vi "log analysis_gps.vi"() -> ()   [LabVIEW 2019] (continued)
0.3968,0.2930,0.5072,0.1078,0.0917,0.0751,0.1476,0.1496,5.0204,0f000001,0*5136ca20\n\t", "INSPVAXA,USB3,0,44.0,FINESTEERING,2107,282107.450,02000000,471d,15824;INS_ALIGNMENT_COMPLETE,INS_RTKFIXED,37.37095551506,126.72370946213,8.7227,22.3000,-0.1464,0.2502,0.0156,-0.936172746,1.990543984,117.627917664,0.3961,0.2929,0.5071,0.1075,0.0916,0.0751,0.1476,0.1496,5.0204,0f000001,0*d8872792\n\t", "INSPVAXA,USB3,0,44.0,FINESTEERING,2107,282107.950,02000000,471d,15824;INS_ALIGNMENT_COMPLETE,INS_RTKFIXED,37.37095481415,126.72371079890,8.7282,22.3000,-0.1478,0.2544,0.0132,-0.866251632,1.815335912,117.612256060,0.3961,0.2929,0.5071,0.1075,0.0916,0.0751,0.1476,0.1496,5.0204,0f000001,0*57d0bda5\n\t", "INSPVAXA,USB3,0,47.5,FINESTEERING,2107,282108.450,02000000,471d,15824;INS_ALIGNMENT_COMPLETE,INS_RTKFIXED,37.37095411436,126.72371215377,8.7320,22.3000,-0.1500,0.2481,0.0140,-1.024789721,1.612981826,117.661458987,0.3956,0.2928,0.5070,0.1077,0.0917,0.0751,0.1475,0.1496,5.0202,0f000001,0*a0675bbc\n\t", "INSPVAXA,USB3,0,47.5,FINESTEERING,2107,282108.950,02000000,471d,15824;INS_ALIGNMENT_COMPLETE,INS_RTKFIXED,37.37095342524,126.72371347450,8.7365,22.3000,-0.1464,0.2522,0.0087,-1.211194385,1.652387786,117.710321786,0.3956,0.2928,0.5070,0.1077,0.0917,0.0751,0.1475,0.1496,5.0202,0f000001,0*fbbb71e9\n\t", "INSPVAXA,USB3,0,48.0,FINESTEERING,2107,282109.450,02000000,471d,15824;INS_ALIGNMENT_COMPLETE,INS_RTKFIXED,37.37095274133,126.72371479106,8.7424,22.3000,-0.1538,0.2512,0.0057,-1.183703798,1.673883858,117.732528128,0.3953,0.2928,0.5071,0.1077,0.0917,0.0751,0.1475,0.1496,5.0195,0f000001,0*a98a5245\n\t", "INSPVAXA,USB3,0,48.0,FINESTEERING,2107,282109.950,02000000,471d,15824;INS_ALIGNMENT_COMPLETE,INS_RTKFIXED,37.37095203304,126.72371616104,8.7487,22.3000,-0.1514,0.2528,0.0147,-1.036882261,1.559922655,117.777953155,0.3953,0.2928,0.5071,0.1077,0.0917,0.0751,0.1475,0.1496,5.0195,0f000001,0*d50cd7f7\n\t", "INSPVAXA,USB3,0,48.5,FINESTEERING,2107,282110.450,02000000,471d,15824;INS_ALIGNMENT_COMPLETE,INS_RTKFIXED,37.37095133527,126.72371748883,8.7530,22.3000,-0.1494,0.2469,0.0119,-1.026348823,1.537323059,117.877652049,0.3951,0.2928,0.5070,0.1077,0.0917,0.0751,0.1475,0.1496,5.0182,0f000001,0*ecbd9d89\n\t", "INSPVAXA,USB3,0,48.5,FINESTEERING,2107,282110.950,02000000,471d,15824;INS_ALIGNMENT_COMPLETE,INS_RTKFIXED,37.37095063141,126.72371883736,8.7567,22.3000,-0.1443,0.2312,0.0129,-1.128303497,1.542678809,118.026662583,0.3951,0.2928,0.5070,0.1077,0.0917,0.0751,0.1475,0.1496,5.0182,0f000001,0*daaca067\n\t", "INSPVAXA,USB3,0,46.0,FINESTEERING,2107,282111.450,02000000,471d,15824;INS_ALIGNMENT_COMPLETE,INS_RTKFIXED,37.37094994978,126.72372015306,8.7620,22.3000,-0.1561,0.2454,0.0089,-1.155550094,1.466986679,118.115120191,0.3996,0.2955,0.5135,0.1085,0.0924,0.0757,0.1476,0.1497,5.0168,0f000001,0*9d755c1d\n\t", "INSPVAXA,USB3,0,46.0,FINESTEERING,2107,282111.950,02000000,471d,15824;INS_ALIGNMENT_COMPLETE,INS_RTKFIXED,37.37094924686,126.72372148621,8.7667,22.3000,-0.1592,0.2411,0.0080,-1.003376747,1.533507787,118.272208873,0.3996,0.2955,0.5135,0.1085,0.0924,0.0757,0.1476,0.1497,5.0168,0f000001,0*68376ab3\n\t", "INSPVAXA,USB3,0,47.5,FINESTEERING,2107,282113.450,02000000,471d,15824;INS_ALIGNMENT_COMPLETE,INS_RTKFIXED,37.37094709383,126.72372548494,8.7822,22.3000,-0.1691,0.2475,0.0112,-0.824972405,1.586356961,118.983770593,0.4030,0.2950,0.5178,0.1084,0.0922,0.0757,0.1475,0.1497,5.0138,0f000001,0*59439988\n\t", "INSPVAXA,USB3,0,51.5,FINESTEERING,2107,282114.950,02000000,471d,15824;INS_ALIGNMENT_COMPLETE,INS_RTKFIXED,37.37094483188,126.72372951627,8.7947,22.3000,-0.1730,0.2314,0.0140,-0.653922567,1.323648308,119.738020967,0.4016,0.2936,0.5159,0.1080,0.0922,0.0755,0.1474,0.1496,5.0125,0f000001,0*093f9180\n\t", "INSPVAXA,USB3,0,50.5,FINESTEERING,2107,282115.450,02000000,471d,15824;INS_ALIGNMENT_COMPLETE,INS_RTKFIXED,37.37094409692,126.72373081199,8.8000,22.3000,-0.1872,0.2511,0.0165,-0.607846314,1.413014132,119.977031024,0.3998,0.2929,0.5140,0.1075,0.0920,0.0753,0.1474,0.1495,5.0103,0f000001,0*d87b3f60\n\t", "INSPVAXA,USB3,0,50.5,FINESTEERING,2107,282115.950,02000000,471d,15824;INS_ALIGNMENT_COMPLETE,INS_RTKFIXED,37.37094333872,126.72373213439,8.8049,22.3000,-0.1750,0.2376,0.0100,-0.458555016,1.505006128,120.195242243,0.3998,0.2929,0.5140,0.1075,0.0920,0.0753,0.1474,0.1495,5.0103,0f000001,0*9085454d\n\t", "INSPVAXA,USB3,0,47.5,FINESTEERING,2107,282116.450,02000000,471d,15824;INS_ALIGNMENT_COMPLETE,INS_RTKFIXED,37.37094260633,126.72373343529,8.8096,22.3000,-0.1820,0.2326,0.0074,-0.394320906,1.730091512,120.395772522,0.3983,0.2926,0.5122,0.1073,0.0921,0.0752,0.1473,0.1495,5.0085,0f000001,0*0af836cc\n\t", "INSPVAXA,USB3,0,47.5,FINESTEERING,2107,282116.950,02000000,471d,15824;INS_ALIGNMENT_COMPLETE,INS_RTKFIXED,37.37094186601,126.72373474956,8.8141,22.3000,-0.1805,0.2419,0.0176,-0.396545512,1.701319201,120.653391507,0.3983,0.2926,0.5122,0.1073,0.0921,0.0752,0.1473,0.1495,5.0085,0f000001,0*1c5a80aa\n\t", "INSPVAXA,USB3,0,50.0,FINESTEERING,2107,282117.450,02000000,471d,15824;INS_ALIGNMENT_COMPLETE,INS_RTKFIXED,37.37094111146,126.72373605556,8.8178,22.3000,-0.1868,0.2460,0.0165,-0.381592646,1.647549493,120.846709462,0.3974,0.2926,0.5106,0.1073,0.0921,0.0751,0.1472,0.1494,5.0066,0f000001,0*ba01e3a8\n\t", "INSPVAXA,USB3,0,50.0,FINESTEERING,2107,282117.950,02000000,471d,15824;INS_ALIGNMENT_COMPLETE,INS_RTKFIXED,37.37094033819,126.72373738098,8.8215,22.3000,-0.1807,0.2431,0.0157,-0.357927005,1.593594515,120.982465037,0.3974,0.2926,0.5106,0.1073,0.0921,0.0751,0.1472,0.1494,5.0066,0f000001,0*473a97aa\n\t", "INSPVAXA,USB3,0,47.0,FINESTEERING,2107,282118.450,02000000,471d,15824;INS_ALIGNMENT_COMPLETE,INS_RTKFIXED,37.37093956964,126.72373870165,8.8242,22.3000,-0.1812,0.2503,0.0145,-0.278070640,1.434405224,121.098239314,0.3976,0.2926,0.5095,0.1073,0.0920,0.0750,0.1472,0.1494,5.0051,0f000001,0*4b2331c4\n\t", "INSPVAXA,USB3,0,47.0,FINESTEERING,2107,282118.950,02000000,471d,15824;INS_ALIGNMENT_COMPLETE,INS_RTKFIXED,37.37093879764,126.72374003076,8.8271,22.3000,-0.1824,0.2531,0.0181,-0.239679007,1.415709773,121.121487507,0.3976,0.2926,0.5095,0.1073,0.0920,0.0750,0.1472,0.1494,5.0051,0f000001,0*31152a6b\n\t", "INSPVAXA,USB3,0,51.0,FINESTEERING,2107,282119.950,02000000,471d,15824;INS_ALIGNMENT_COMPLETE,INS_RTKFIXED,37.37093727154,126.72374264951,8.8356,22.3000,-0.1820,0.2425,0.0126,-0.263751885,1.526286422,121.184806545,0.3974,0.2926,0.5086,0.1074,0.0920,0.0750,0.1471,0.1494,5.0040,0f000001,0*c7b594c4\n\t", "INSPVAXA,USB3,0,49.5,FINESTEERING,2107,282121.950,02000000,471d,15824;INS_ALIGNMENT_COMPLETE,INS_RTKFIXED,37.37093422508,126.72374790381,8.8513,22.3000,-0.1769,0.2415,0.0095,-0.361327537,1.582717888,121.199299020,0.3976,0.2927,0.5074,0.1074,0.0918,0.0750,0.1470,0.1494,5.0032,0f000001,0*bd59e65f\n\t", "INSPVAXA,USB3,0,51.5,FINESTEERING,2107,282122.950,02000000,471d,15824;INS_ALIGNMENT_COMPLETE,INS_RTKFIXED,37.37093271089,126.72375052599,8.8596,22.3000,-0.1652,0.2321,0.0060,-0.281890113,1.847721307,121.184840630,0.3974,0.2927,0.5070,0.1074,0.0918,0.0750,0.1469,0.1494,5.0040,0f000001,0*3de7c804\n\t", "INSPVAXA,USB3,0,51.0,FINESTEERING,2107,282151.500,02000000,471d,15824;INS_ALIGNMENT_COMPLETE,INS_RTKFIXED,37.37088960505,126.72382499990,9.1778,22.3000,-0.1858,0.2425,0.0007,-0.584217482,1.708777597,119.499420224,0.4348,0.2933,0.5266,0.1137,0.0921,0.0762,0.1458,0.1498,5.0245,0f000001,0*a137cdab\n\t", "INSPVAXA,USB3,0,46.5,FINESTEERING,2107,282153.500,02000000,471d,15824;INS_ALIGNMENT_COMPLETE,INS_RTKFIXED,37.37088668027,126.72383030308,9.1844,22.3000,-0.1846,0.2433,-0.0063,-0.490970731,1.271254139,120.414068071,0.4478,0.2935,0.5351,0.1145,0.0921,0.0767,0.1457,0.1497,5.0277,0f000001,0*2a0513c3\n\t", "INSPVAXA,USB3,0,47.0,FINESTEERING,2107,282154.500,02000000,471d,15824;INS_ALIGNMENT_COMPLETE,INS_RTKFIXED,37.37088518540,126.72383296501,9.1848,22.3000,-0.1849,0.2389,0.0033,-0.578089293,1.343840193,120.921980586,0.4509,0.2935,0.5383,0.1145,0.0921,0.0767,0.1457,0.1497,5.0293,0f000001,0*6c2251c0\n\t", "INSPVAXA,USB3,0,49.5,FINESTEERING,2107,282156.000,02000000,471d,15824;INS_ALIGNMENT_COMPLETE,INS_RTKFIXED,37.37088292743,126.72383688922,9.1933,22.3000,-0.1804,0.2249,-0.0069,-0.526000833,1.617795510,121.650926042,0.4526,0.2935,0.5409,0.1144,0.0920,0.0768,0.1457,0.1496,5.0309,0f000001,0*7b06a300\n\t", "INSPVAXA,USB3,0,48.5,FINESTEERING,2107,282156.500,02000000,471d,15824;INS_ALIGNMENT_COMPLETE,INS_RTKFIXED,37.37088217363,126.72383817131,9.1964,22.3000,-0.1807,0.2394,-0.0085,-0.574321613,1.643212102,121.914347439,0.4534,0.2936,0.5427,0.1143,0.0921,0.0768,0.1456,0.1496,5.0325,0f000001,0*15ca3725\n\t", "INSPVAXA,USB3,0,48.5,FINESTEERING,2107,282157.000,02000000,471d,15824;INS_ALIGNMENT_COMPLETE,INS_RTKFIXED,37.37088140399,126.72383945930,9.1993,22.3000,-0.1862,0.2446,-0.0064,-0.600405217,1.496036608,122.180467270,0.4534,0.2936,0.5427,0.1143,0.0921,0.0768,0.1456,0.1496,5.0325,0f000001,0*c5e5c6e3\n\t", "INSPVAXA,USB3,0,45.5,FINESTEERING,2107,282158.500,02000000,471d,15824;INS_ALIGNMENT_COMPLETE,INS_RTKFIXED,37.37087907876,126.72384326761,9.2104,22.3000,-0.1767,0.2291,0.0108,-0.395230088,1.351210238,122.917750135,0.4537,0.2937,0.5451,0.1144,0.0921,0.0768,0.1456,0.1495,5.0357,0f000001,0*07daf6c2\n\t", "INSPVAXA,USB3,0,45.5,FINESTEERING,2107,282159.000,02000000,471d,15824;INS_ALIGNMENT_COMPLETE,INS_RTKFIXED,37.37087827658,126.72384453527,9.2150,22.3000,-0.1825,0.2336,0.0127,-0.281125763,1.400376320,123.162742277,0.4537,0.2937,0.5451,0.1144,0.0921,0.0768,0.1456,0.1495,5.0357,0f000001,0*5700aa0a\n\t", "INSPVAXA,USB3,0,48.5,FINESTEERING,2107,282161.000,02000000,471d,15824;INS_ALIGNMENT_COMPLETE,INS_RTKFIXED,37.37087514986,126.72384964420,9.2386,22.3000,-0.1845,0.2318,0.0206,-0.134311793,1.526790970,123.449672080,0.4533,0.2938,0.5460,0.1147,0.0921,0.0768,0.1455,0.1496,5.0387,0f000001,0*1e397fdc\n\t", "INSPVAXA,USB3,0,49.0,FINESTEERING,2107,282162.000,02000000,471d,15824;INS_ALIGNMENT_COMPLETE,INS_RTKFIXED,37.37087356615,126.72385221886,9.2529,22.3000,-0.1851,0.2394,-0.0036,-0.080021339,1.630723538,123.455447603,0.4532,0.2939,0.5462,0.1148,0.0921,0.0768,0.1454,0.1496,5.0402,0f000001,0*5854c212\n\t", "INSPVAXA,USB3,0,51.0,FINESTEERING,2107,282162.500,02000000,471d,15824;INS_ALIGNMENT_COMPLETE,INS_RTKFIXED,37.37087276598,126.72385350535,9.2616,22.3000,-0.1911,0.2293,0.0115,-0.073182754,1.698964868,123.450820933,0.4532,0.2939,0.5462,0.1150,0.0921,0.0768,0.1454,0.1496,5.0417,0f000001,0*35a5fbef\n\t", "INSPVAXA,USB3,0,51.0,FINESTEERING,2107,282163.000,02000000,471d,15824;INS_ALIGNMENT_COMPLETE,INS_RTKFIXED,37.37087198418,126.72385476769,9.2713,22.3000,-0.1886,0.2265,0.0207,-0.163897307,1.756288597,123.387194402,0.4532,0.2939,0.5462,0.1150,0.0921,0.0768,0.1454,0.1496,5.0417,0f000001,0*f7296fb4\n\t", "INSPVAXA,USB3,0,50.0,FINESTEERING,2107,282163.500,02000000,471d,15824;INS_ALIGNMENT_COMPLETE,INS_RTKFIXED,37.37087116734,126.72385603736,9.2795,22.3000,-0.1822,0.2264,0.0180,-0.228587283,1.950230328,123.198406451,0.4532,0.2939,0.5462,0.1150,0.0921,0.0768,0.1454,0.1496,5.0417,0f000001,0*1ae1e07b\n\t", "INSPVAXA,USB3,0,50.0,FINESTEERING,2107,282164.000,02000000,471d,15824;INS_ALIGNMENT_COMPLETE,INS_RTKFIXED,37.37087034978,126.72385731621,9.2879,22.3000,-0.1896,0.2295,0.0123,-0.289631727,1.840561194,122.888440752,0.4532,0.2939,0.5462,0.1150,0.0921,0.0768,0.1454,0.1496,5.0417,0f000001,0*056b33eb\n\t", "INSPVAXA,USB3,0,49.5,FINESTEERING,2107,282164.500,02008000,471d,15824;INS_ALIGNMENT_COMPLETE,INS_RTKFIXED,37.37086961397,126.72385855899,9.2957,22.3000,-0.1725,0.2178,0.0037,-0.245083318,1.835832496,122.519490120,0.5068,0.3317,0.5928,0.1224,0.0977,0.0793,0.1462,0.1507,5.0448,0f000001,0*242e4928\n\t", "INSPVAXA,USB3,0,49.5,FINESTEERING,2107,282165.000,02008000,471d,15824;INS_ALIGNMENT_COMPLETE,INS_RTKFIXED,37.37086887660,126.72385979146,9.3053,22.3000,-0.1797,0.2392,0.0086,-0.083873160,1.728047221,122.128251979,0.5068,0.3317,0.5928,0.1224,0.0977,0.0793,0.1462,0.1507,5.0448,0f000001,0*7f8693c0\n\t", "INSPVAXA,USB3,0,50.0,FINESTEERING,2107,282165.500,02008000,471d,15824;INS_ALIGNMENT_COMPLETE,INS_RTKFIXED,37.37086811316,126.72386104230,9.3143,22.3000,-0.1621,0.2209,0.0106,0.024861587,1.649578148,121.656445407,0.4863,0.3145,0.5830,0.1190,0.0946,0.0782,0.1458,0.1502,5.0461,0f000001,0*34f23d42\n\t", "INSPVAXA,USB3,0,50.0,FINESTEERING,2107,282166.000,02008000,471d,15824;INS_ALIGNMENT_COMPLETE,INS_RTKFIXED,37.37086751829,126.72386195729,9.3219,22.3000,-0.0093,-0.0451,0.0007,-0.021903893,1.492441336,121.617580212,0.4863,0.3145,0.5830,0.1190,0.0946,0.0782,0.1458,0.1502,5.0461,0f000001,0*e5b24ae3\n\t", "INSPVAXA,USB3,0,48.5,FINESTEERING,2107,282166.500,02008000,471d,15824;INS_ALIGNMENT_COMPLETE,INS_RTKFIXED,37.37086745954,126.72386181526,9.3232,22.3000,-0.0268,-0.0236,0.0089,-0.043372783,1.566427448,121.563343894,0.4732,0.3047,0.5748,0.1189,0.0947,0.0774,0.1456,0.1500,5.0475,0f000001,0*3570ed60\n\t", "INSPVAXA,USB3,0,48.5,FINESTEERING,2107,282167.000,02008000,471d,15824;INS_ALIGNMENT_COMPLETE,INS_RTKFIXED,37.37086722262,126.72386202898,9.3264,22.3000,-0.1700,0.2085,0.0159,-0.059764704,1.681922525,121.297414016,0.4732,0.3047,0.5748,0.1189,0.0947,0.0774,0.1456,0.1500,5.0475,0f000001,0*686f29fa\n\t", "INSPVAXA,USB3,0,51.0,FINESTEERING,2107,282167.500,02008000,471d,15824;INS_ALIGNMENT_COMPLETE,INS_RTKFIXED,37.37086635075,126.72386343693,9.3355,22.3000,-0.1343,0.1551,0.0138,-0.191041256,1.725233794,121.448181107,0.4732,0.3047,0.5748,0.1189,0.0947,0.0774,0.1456,0.1500,5.0475,0f000001,0*c09661b1\n\t", "INSPVAXA,USB3,0,51.0,FINESTEERING,2107,282168.000,02008000,471d,15824;INS_ALIGNMENT_COMPLETE,INS_RTKFIXED,37.37086554629,126.72386469627,9.3449,22.3000,-0.1443,0.1947,0.0175,-0.193885511,1.717406727,121.172307594,0.4732,0.3047,0.5748,0.1189,0.0947,0.0774,0.1456,0.1500,5.0475,0f000001,0*05ac97bf\n\t", "INSPVAXA,USB3,0,51.0,FINESTEERING,2107,282168.500,02000000,471d,15824;INS_ALIGNMENT_COMPLETE,INS_RTKFIXED,37.37086484906,126.72386602613,9.3508,22.3000,-0.1684,0.2118,0.0292,-0.052015142,1.767687292,120.756942814,0.5200,0.3367,0.6136,0.1257,0.1009,0.0794,0.1465,0.1509,5.0427,0f000001,0*74b10fb1\n\t", "INSPVAXA,USB3,0,51.0,FINESTEERING,2107,282169.000,02000000,471d,15824;INS_ALIGNMENT_COMPLETE,INS_RTKFIXED,37.37086415822,126.72386736868,9.3575,22.3000,-0.1707,0.2211,0.0151,0.018670150,1.718273405,120.397652354,0.5200,0.3367,0.6136,0.1257,0.1009,0.0794,0.1465,0.1509,5.0427,0f000001,0*7f0a75ca\n\t", "INSPVAXA,USB3,0,46.0,FINESTEERING,2107,282169.500,02000000,471d,15824;INS_ALIGNMENT_COMPLETE,INS_RTKFIXED,37.37086344397,126.72386871844,9.3630,22.3000,-0.1742,0.2275,0.0011,-0.016191041,1.633927809,119.983496476,0.4955,0.3175,0.5974,0.1215,0.0969,0.0780,0.1460,0.1504,5.0326,0f000001,0*70440743\n\t", "DUALANTENNAHEADINGA,USB3,0,46.0,FINESTEERING,2107,282170.000,02000000,d426,15824;INSUFFICIENT_OBS,NONE,0.000000000,0.000000000,0.000000000,0.0,0.000000000,0.000000000,\"\",0,0,0,0,00,00,00,00*d9bd9ff7\n\t", "INSPVAXA,USB3,0,49.5,FINESTEERING,2107,282170.500,02000000,471d,15824;INS_ALIGNMENT_COMPLETE,INS_RTKFIXED,37.37086196149,126.72387133593,9.3775,22.3000,-0.1638,0.2319,0.0101,-0.134678922,1.597363801,119.344832889,0.4955,0.3175,0.5974,0.1215,0.0969,0.0780,0.1460,0.1504,5.0326,0f000001,0*0ad13adf\n\t", "INSPVAXA,USB3,0,49.5,FINESTEERING,2107,282171.000,02000000,471d,15824;INS_ALIGNMENT_COMPLETE,INS_RTKFIXED,37.37086118756,126.72387260380,9.3866,22.3000,-0.1780,0.2223,0.0226,-0.237576400,1.617402983,119.136823599,0.4955,0.3175,0.5974,0.1215,0.0969,0.0780,0.1460,0.1504,5.0326,0f000001,0*d3c2583e\n\t", "DUALANTENNAHEADINGA,USB3,0,52.5,FINESTEERING,2107,282171.500,02000000,d426,15824;SOL_COMPUTED,L1_FLOAT,-1.000000000,212.575851440,56.383117676,0.0,44.713680267,134.992919922,\"631T\",11,5,5,5,04,00,20,02*bb8370c9\n\t", "INSPVAXA,USB3,0,52.5,FINESTEERING,2107,282172.000,02000000,471d,15824;INS_ALIGNMENT_COMPLETE,INS_RTKFIXED,37.37085961658,126.72387509904,9.4055,22.3000,-0.1866,0.2197,0.0120,-0.164173617,1.908755927,118.881251858,0.4955,0.3175,0.5974,0.1215,0.0969,0.0780,0.1460,0.1504,5.0326,0f000001,0*7b1cb490\n\t", "DUALANTENNAHEADINGA,USB3,0,51.0,FINESTEERING,2107,282172.500,02008000,d426,15824;SOL_COMPUTED,NARROW_FLOAT,-1.000000000,128.001327515,-71.010498047,0.0,360.000000000,151.438781738,\"631T\",13,7,7,5,04,00,20,03*76c36059\n\t", "INSPVAXA,USB3,0,51.0,FINESTEERING,2107,282173.000,02008000,471d,15824;INS_ALIGNMENT_COMPLETE,INS_RTKFIXED,37.37085833527,126.72387797741,9.4066,22.3000,-0.1810,0.2279,0.0198,-0.406869052,2.030704243,118.923772886,0.5770,0.3723,0.6754,0.1336,0.1058,0.0814,0.1476,0.1521,5.0145,0f000001,0*4f67786d\n\t", "INSPVAXA,USB3,0,51.0,FINESTEERING,2107,282173.500,02008000,471d,15824;INS_ALIGNMENT_COMPLETE,INS_RTKFIXED,37.37085763620,126.72387935658,9.4103,22.3000,-0.1736,0.2330,0.0207,-0.517446305,1.873578132,118.931812586,0.5249,0.3329,0.6407,0.1266,0.1009,0.0786,0.1470,0.1512,5.0071,0f000001,0*4ebf01a6\n\t", "DUALANTENNAHEADINGA,USB3,0,51.0,FINESTEERING,2107,282174.000,02008000,d426,15824;SOL_COMPUTED,NARROW_FLOAT,-1.000000000,123.069808960,-65.629364014,0.0,360.000000000,180.000000000,\"631T\",16,6,6,5,04,00,20,03*92b169c2\n\t", "DUALANTENNAHEADINGA,USB3,0,49.0,FINESTEERING,2107,282174.500,02008000,d426,15824;SOL_COMPUTED,NARROW_FLOAT,-1.000000000,124.551315308,-68.632659912,0.0,360.000000000,180.000000000,\"631T\",16,7,7,5,04,00,20,03*6a9e420e\n\t", "INSPVAXA,USB3,0,49.0,FINESTEERING,2107,282175.000,02008000,471d,15824;INS_ALIGNMENT_COMPLETE,INS_RTKFIXED,37.37085549477,126.72388337891,9.4209,22.3000,-0.1860,0.2237,0.0201,-0.564638995,1.417085276,119.025707092,0.4961,0.3139,0.6151,0.1240,0.1000,0.0771,0.1467,0.1509,5.0036,0f000001,0*2746038f\n\t", "INSPVAXA,USB3,0,50.0,FINESTEERING,2107,282175.500,02008000,471d,15824;INS_ALIGNMENT_COMPLETE,INS_RTKFIXED,37.37085479315,126.72388469742,9.4248,22.3000,-0.1822,0.2271,0.0141,-0.513806522,1.414717204,119.104354508,0.4791,0.3046,0.5957,0.1234,0.0999,0.0764,0.1464,0.1507,5.0029,0f000001,0*e3204e40\n\t", "INSPVAXA,USB3,0,50.0,FINESTEERING,2107,282176.000,02008000,471d,15824;INS_ALIGNMENT_COMPLETE,INS_RTKFIXED,37.37085410326,126.72388599341,9.4283,22.3000,-0.1760,0.2106,0.0151,-0.605541417,1.454743259,119.281713752,0.4791,0.3046,0.5957,0.1234,0.0999,0.0764,0.1464,0.1507,5.0029,0f000001,0*bcb93fc8\n\t", "DUALANTENNAHEADINGA,USB3,0,48.5,FINESTEERING,2107,282176.500,02000000,d426,15824;SOL_COMPUTED,NARROW_FLOAT,-1.000000000,134.305130005,-57.419616699,0.0,360.000000000,180.000000000,\"631T\",18,6,6,5,04,00,20,03*ffb18b5f\n\t", "DUALANTENNAHEADINGA,USB3,0,48.5,FINESTEERING,2107,282177.000,02000000,d426,15824;SOL_COMPUTED,NARROW_FLOAT,-1.000000000,135.311111450,-57.297637939,0.0,360.000000000,180.000000000,\"631T\",18,6,6,5,04,00,20,03*ffb49dec\n\t", "INSPVAXA,USB3,0,48.0,FINESTEERING,2107,282177.500,02000000,471d,15824;INS_ALIGNMENT_COMPLETE,INS_RTKFIXED,37.37085188860,126.72389002075,9.4437,22.3000,-0.1883,0.2420,0.0164,-0.505003517,1.427423679,120.083460934,0.4645,0.2990,0.5702,0.1231,0.0988,0.0761,0.1455,0.1502,5.0044,0f000001,0*390fa34e\n\t", "INSPVAXA,USB3,0,48.0,FINESTEERING,2107,282178.000,02000000,471d,15824;INS_ALIGNMENT_COMPLETE,INS_RTKFIXED,37.37085112539,126.72389137243,9.4485,22.3000,-0.1737,0.2237,0.0239,-0.447467240,1.418285202,120.360306359,0.4645,0.2990,0.5702,0.1231,0.0988,0.0761,0.1455,0.1502,5.0044,0f000001,0*ee66b8d3\n\t", "DUALANTENNAHEADINGA,USB3,0,48.5,FINESTEERING,2107,282178.500,02000000,d426,15824;SOL_COMPUTED,L1_FLOAT,-1.000000000,214.039077759,54.311355591,0.0,31.311414719,120.360610962,\"631T\",17,5,5,5,04,00,20,02*7f9a84dc\n\t", "INSPVAXA,USB3,0,48.5,FINESTEERING,2107,282179.000,02000000,471d,15824;INS_ALIGNMENT_COMPLETE,INS_RTKFIXED,37.37084962670,126.72389402617,9.4575,22.3000,-0.1964,0.2240,0.0138,-0.716798061,1.635103136,120.928637388,0.4619,0.2984,0.5621,0.1226,0.0976,0.0763,0.1451,0.1499,5.0052,0f000001,0*33d16cf5\n\t", "INSPVAXA,USB3,0,50.0,FINESTEERING,2107,282179.500,02000000,471d,15824;INS_ALIGNMENT_COMPLETE,INS_RTKFIXED,37.37084886052,126.72389534484,9.4614,22.3000,-0.1928,0.2247,0.0047,-0.502133863,1.643703431,121.221936688,0.4606,0.2980,0.5561,0.1219,0.0962,0.0765,0.1448,0.1496,5.0057,0f000001,0*d5b8afd0\n\t", "INSPVAXA,USB3,0,50.0,FINESTEERING,2107,282180.000,02000000,471d,15824;INS_ALIGNMENT_COMPLETE,INS_RTKFIXED,37.37084808459,126.72389666090,9.4649,22.3000,-0.1925,0.2192,0.0119,-0.378680064,1.659778733,121.498244377,0.4606,0.2980,0.5561,0.1219,0.0962,0.0765,0.1448,0.1496,5.0057,0f000001,0*ef9263b5\n\t", "DUALANTENNAHEADINGA,USB3,0,50.0,FINESTEERING,2107,282180.500,02000000,d426,15824;INSUFFICIENT_OBS,NONE,0.000000000,0.000000000,0.000000000,0.0,0.000000000,0.000000000,\"\",0,0,0,0,00,00,00,00*7c3513f7\n\t", "DUALANTENNAHEADINGA,USB3,0,50.0,FINESTEERING,2107,282181.000,02000000,d426,15824;INSUFFICIENT_OBS,NONE,0.000000000,0.000000000,0.000000000,0.0,0.000000000,0.000000000,\"\",0,0,0,0,00,00,00,00*d5a670f0\n\t", "DUALANTENNAHEADINGA,USB3,0,51.0,FINESTEERING,2107,282181.500,02000000,d426,15824;SOL_COMPUTED,L1_FLOAT,-1.000000000,135.320739746,-67.288024902,0.0,360.000000000,180.000000000,\"631T\",16,6,6,4,04,00,20,03*b9d4ea0f\n\t", "DUALANTENNAHEADINGA,USB3,0,51.0,FINESTEERING,2107,282182.000,02000000,d426,15824;SOL_COMPUTED,L1_FLOAT,-1.000000000,135.798538208,-66.526153564,0.0,360.000000000,180.000000000,\"631T\",19,6,6,3,04,00,20,00*2967dc6a\n\t", "INSPVAXA,USB3,0,49.0,FINESTEERING,2107,282182.500,02000000,471d,15824;INS_ALIGNMENT_COMPLETE,INS_RTKFIXED,37.37084393721,126.72390297520,9.4968,22.3000,-0.2002,0.2134,0.0137,-0.651107521,1.170361863,122.939925996,0.5624,0.3670,0.6434,0.1330,0.1041,0.0813,0.1464,0.1511,5.0059,0f000001,0*617b26b7\n\t", "DUALANTENNAHEADINGA,USB3,0,49.0,FINESTEERING,2107,282183.000,02000000,d426,15824;INSUFFICIENT_OBS,NONE,0.000000000,0.000000000,0.000000000,0.0,0.000000000,0.000000000,\"\",0,0,0,0,00,00,00,00*b274769d\n\t", "DUALANTENNAHEADINGA,USB3,0,47.0,FINESTEERING,2107,282183.500,02000000,d426,15824;INSUFFICIENT_OBS,NONE,0.000000000,0.000000000,0.000000000,0.0,0.000000000,0.000000000,\"\",0,0,0,0,00,00,00,00*9278fa5b\n\t", "DUALANTENNAHEADINGA,USB3,0,47.0,FINESTEERING,2107,282184.000,02000000,d426,15824;INSUFFICIENT_OBS,NONE,0.000000000,0.000000000,0.000000000,0.0,0.000000000,0.000000000,\"\",0,0,0,0,00,00,00,00*4a16a1eb\n\t", "DUALANTENNAHEADINGA,USB3,0,49.0,FINESTEERING,2107,282184.500,02000000,d426,15824;SOL_COMPUTED,NARROW_FLOAT,-1.000000000,146.879547119,-70.479187012,0.0,360.000000000,121.135261536,\"631T\",18,7,7,5,04,00,20,03*9a26e641\n\t", "DUALANTENNAHEADINGA,USB3,0,49.0,FINESTEERING,2107,282185.000,02000000,d426,15824;SOL_COMPUTED,NARROW_FLOAT,-1.000000000,146.221954346,-70.420104980,0.0,360.000000000,123.181526184,\"631T\",18,7,7,5,04,00,20,03*8e5bbb52\n\t", "DUALANTENNAHEADINGA,USB3,0,46.5,FINESTEERING,2107,282185.500,02000000,d426,15824;INSUFFICIENT_OBS,NONE,0.000000000,0.000000000,0.000000000,0.0,0.000000000,0.000000000,\"\",0,0,0,0,00,00,00,00*a89f4c07\n\t", "INSPVAXA,USB3,0,46.5,FINESTEERING,2107,282186.000,02000000,471d,15824;INS_ALIGNMENT_COMPLETE,INS_RTKFIXED,37.37083829479,126.72391206471,9.5210,22.3000,-0.2075,0.2040,0.0190,-0.387614347,1.152152032,123.294354417,0.6060,0.3885,0.7100,0.1370,0.1076,0.0827,0.1473,0.1517,5.0026,0f000001,0*983cddfa\n\t", "DUALANTENNAHEADINGA,USB3,0,50.5,FINESTEERING,2107,282186.500,02000000,d426,15824;INSUFFICIENT_OBS,NONE,0.000000000,0.000000000,0.000000000,0.0,0.000000000,0.000000000,\"\",0,0,0,0,00,00,00,00*e63b13e8\n\t", "INSPVAXA,USB3,0,50.5,FINESTEERING,2107,282187.000,02000000,471d,15824;INS_ALIGNMENT_COMPLETE,INS_RTKFIXED,37.37083651711,126.72391453390,9.5369,22.3000,-0.1989,0.2174,0.0087,-0.266896449,1.151079764,122.361675094,0.6060,0.3885,0.7100,0.1370,0.1076,0.0827,0.1473,0.1517,5.0026,0f000001,0*c07c766a\n\t", "DUALANTENNAHEADINGA,USB3,0,50.0,FINESTEERING,2107,282187.500,02000000,d426,15824;INSUFFICIENT_OBS,NONE,0.000000000,0.000000000,0.000000000,0.0,0.000000000,0.000000000,\"\",0,0,0,0,00,00,00,00*f7dadc56\n\t", "DUALANTENNAHEADINGA,USB3,0,50.0,FINESTEERING,2107,282188.000,02000000,d426,15824;INSUFFICIENT_OBS,NONE,0.000000000,0.000000000,0.000000000,0.0,0.000000000,0.000000000,\"\",0,0,0,0,00,00,00,00*92e72652\n\t", "DUALANTENNAHEADINGA,USB3,0,53.5,FINESTEERING,2107,282188.500,02000000,d426,15824;INSUFFICIENT_OBS,NONE,0.000000000,0.000000000,0.000000000,0.0,0.000000000,0.000000000,\"\",0,0,0,0,00,00,00,00*10de566f\n\t", "DUALANTENNAHEADINGA,USB3,0,53.5,FINESTEERING,2107,282189.000,02000000,d426,15824;INSUFFICIENT_OBS,NONE,0.000000000,0.000000000,0.000000000,0.0,0.000000000,0.000000000,\"\",0,0,0,0,00,00,00,00*b94d3568\n\t", "DUALANTENNAHEADINGA,USB3,0,51.5,FINESTEERING,2107,282189.500,02000000,d426,15824;INSUFFICIENT_OBS,NONE,0.000000000,0.000000000,0.000000000,0.0,0.000000000,0.000000000,\"\",0,0,0,0,00,00,00,00*706ecbbe\n\t", "DUALANTENNAHEADINGA,USB3,0,51.5,FINESTEERING,2107,282190.000,02000000,d426,15824;INSUFFICIENT_OBS,NONE,0.000000000,0.000000000,0.000000000,0.0,0.000000000,0.000000000,\"\",0,0,0,0,00,00,00,00*9080aeab\n\t", "DUALANTENNAHEADINGA,USB3,0,51.5,FINESTEERING,2107,282190.500,02000000,d426,15824;SOL_COMPUTED,NARROW_FLOAT,-1.000000000,135.085830688,-53.305603027,0.0,360.000000000,180.000000000,\"631T\",17,6,6,5,04,00,20,03*0a25629d\n\t", "DUALANTENNAHEADINGA,USB3,0,51.5,FINESTEERING,2107,282191.000,02000000,d426,15824;SOL_COMPUTED,NARROW_FLOAT,-1.000000000,135.135757446,-54.312408447,0.0,360.000000000,180.000000000,\"631T\",18,6,6,5,04,00,20,03*2fbb2179\n\t", "DUALANTENNAHEADINGA,USB3,0,51.0,FINESTEERING,2107,282191.500,02000000,d426,15824;SOL_COMPUTED,NARROW_FLOAT,-1.000000000,134.974884033,-69.401855469,0.0,360.000000000,164.567916870,\"631T\",18,7,7,5,04,00,20,03*c918ed4a\n\t", "DUALANTENNAHEADINGA,USB3,0,51.0,FINESTEERING,2107,282192.000,02000000,d426,15824;SOL_COMPUTED,NARROW_FLOAT,-1.000000000,134.756271362,-69.514831543,0.0,360.000000000,164.104385376,\"631T\",19,7,7,5,04,00,20,03*4a4dea82\n\t", "DUALANTENNAHEADINGA,USB3,0,48.5,FINESTEERING,2107,282192.500,02000000,d426,15824;INSUFFICIENT_OBS,NONE,0.000000000,0.000000000,0.000000000,0.0,0.000000000,0.000000000,\"\",0,0,0,0,00,00,00,00*a4d33cd7\n\t", "DUALANTENNAHEADINGA,USB3,0,48.5,FINESTEERING,2107,282193.000,02000000,d426,15824;INSUFFICIENT_OBS,NONE,0.000000000,0.000000000,0.000000000,0.0,0.000000000,0.000000000,\"\",0,0,0,0,00,00,00,00*0d405fd0\n\t", "DUALANTENNAHEADINGA,USB3,0,50.5,FINESTEERING,2107,282193.500,02000000,d426,15824;SOL_COMPUTED,NARROW_FLOAT,-1.000000000,151.214721680,75.840576172,0.0,311.274841309,57.009273529,\"631T\",15,8,8,5,04,00,20,03*7af4d743\n\t", "DUALANTENNAHEADINGA,USB3,0,50.5,FINESTEERING,2107,282194.000,02000000,d426,15824;SOL_COMPUTED,NARROW_FLOAT,-1.000000000,150.594802856,75.862449646,0.0,315.079772949,56.983615875,\"631T\",15,8,8,5,04,00,20,03*a31139df\n\t", "DUALANTENNAHEADINGA,USB3,0,49.5,FINESTEERING,2107,282194.500,02008000,d426,15824;SOL_COMPUTED,NARROW_FLOAT,-1.000000000,75.730995178,-6.270477295,0.0,224.747741699,180.000000000,\"631T\",15,8,8,5,04,00,20,03*aae5cd6a\n\t", "DUALANTENNAHEADINGA,USB3,0,49.5,FINESTEERING,2107,282195.000,02008000,d426,15824;SOL_COMPUTED,NARROW_FLOAT,-1.000000000,76.029739380,-7.977203369,0.0,225.982131958,180.000000000,\"631T\",16,8,8,5,04,00,20,03*1aef0704\n\t", "DUALANTENNAHEADINGA,USB3,0,50.0,FINESTEERING,2107,282195.500,02008000,d426,15824;INSUFFICIENT_OBS,NONE,0.000000000,0.000000000,0.000000000,0.0,0.000000000,0.000000000,\"\",0,0,0,0,00,00,00,00*3a754bb7\n\t", "DUALANTENNAHEADINGA,USB3,0,50.0,FINESTEERING,2107,282196.000,02008000,d426,15824;INSUFFICIENT_OBS,NONE,0.000000000,0.000000000,0.000000000,0.0,0.000000000,0.000000000,\"\",0,0,0,0,00,00,00,00*bcb2c0dd\n\t", "DUALANTENNAHEADINGA,USB3,0,49.0,FINESTEERING,2107,282196.500,02008000,d426,15824;SOL_COMPUTED,NARROW_FLOAT,-1.000000000,119.397575378,5.704736233,0.0,360.000000000,180.000000000,\"631T\",17,6,6,5,04,00,20,03*618b4b70\n\t", "DUALANTENNAHEADINGA,USB3,0,52.0,FINESTEERING,2107,282197.500,02008000,d426,15824;SOL_COMPUTED,NARROW_FLOAT,-1.000000000,59.046657562,-17.785888672,0.0,166.409759521,180.000000000,\"631T\",16,7,7,5,04,00,20,03*00118b7f\n\t", "DUALANTENNAHEADINGA,USB3,0,52.0,FINESTEERING,2107,282198.000,02008000,d426,15824;SOL_COMPUTED,NARROW_FLOAT,-1.000000000,59.079334259,-18.122131348,0.0,167.196258545,180.000000000,\"631T\",16,7,7,5,04,00,20,03*485efbcb\n\t", "DUALANTENNAHEADINGA,USB3,0,50.0,FINESTEERING,2107,282198.500,02000000,d426,15824;SOL_COMPUTED,NARROW_FLOAT,-1.000000000,72.630279541,-6.125091553,0.0,217.219696045,180.000000000,\"631T\",16,8,8,5,04,00,20,03*03cea49d\n\t", "DUALANTENNAHEADINGA,USB3,0,50.0,FINESTEERING,2107,282199.000,02000000,d426,15824;SOL_COMPUTED,NARROW_FLOAT,-1.000000000,72.616973877,-5.097595215,0.0,218.517272949,180.000000000,\"631T\",18,8,8,5,04,00,20,03*278af582\n\t", "DUALANTENNAHEADINGA,USB3,0,51.0,FINESTEERING,2107,282199.500,02000000,d426,15824;INSUFFICIENT_OBS,NONE,0.000000000,0.000000000,0.000000000,0.0,0.000000000,0.000000000,\"\",0,0,0,0,00,00,00,00*6fb354b0\n\t", "DUALANTENNAHEADINGA,USB3,0,51.5,FINESTEERING,2107,282200.500,02000000,d426,15824;INSUFFICIENT_OBS,NONE,0.000000000,0.000000000,0.000000000,0.0,0.000000000,0.000000000,\"\",0,0,0,0,00,00,00,00*ba5dc1a6\n\t", "DUALANTENNAHEADINGA,USB3,0,51.5,FINESTEERING,2107,282201.000,02000000,d426,15824;INSUFFICIENT_OBS,NONE,0.000000000,0.000000000,0.000000000,0.0,0.000000000,0.000000000,\"\",0,0,0,0,00,00,00,00*13cea2a1\n\t", "DUALANTENNAHEADINGA,USB3,0,53.0,FINESTEERING,2107,282201.500,02000000,d426,15824;INSUFFICIENT_OBS,NONE,0.000000000,0.000000000,0.000000000,0.0,0.000000000,0.000000000,\"\",0,0,0,0,00,00,00,00*311e64df\n\t", "INSPVAXA,USB3,0,53.0,FINESTEERING,2107,282202.050,02000000,471d,15824;INS_ALIGNMENT_COMPLETE,INS_RTKFIXED,37.37081327952,126.72395394538,9.6368,22.3000,-0.2188,0.2169,0.0119,-0.186356861,0.873042918,124.050200417,0.5705,0.3686,0.6665,0.1331,0.1050,0.0820,0.1461,0.1508,4.9895,0f000001,0*b1c71fb3\n\t", "DUALANTENNAHEADINGA,USB3,0,53.0,FINESTEERING,2107,282202.500,02000000,d426,15824;INSUFFICIENT_OBS,NONE,0.000000000,0.000000000,0.000000000,0.0,0.000000000,0.000000000,\"\",0,0,0,0,00,00,00,00*e4587ba4\n\t", "DUALANTENNAHEADINGA,USB3,0,52.5,FINESTEERING,2107,282203.500,02000000,d426,15824;INSUFFICIENT_OBS,NONE,0.000000000,0.000000000,0.000000000,0.0,0.000000000,0.000000000,\"\",0,0,0,0,00,00,00,00*55500259\n\t", "DUALANTENNAHEADINGA,USB3,0,52.5,FINESTEERING,2107,282204.000,02000000,d426,15824;INSUFFICIENT_OBS,NONE,0.000000000,0.000000000,0.000000000,0.0,0.000000000,0.000000000,\"\",0,0,0,0,00,00,00,00*8d3e59e9\n\t", "DUALANTENNAHEADINGA,USB3,0,51.0,FINESTEERING,2107,282204.500,02000000,d426,15824;INSUFFICIENT_OBS,NONE,0.000000000,0.000000000,0.000000000,0.0,0.000000000,0.000000000,\"\",0,0,0,0,00,00,00,00*0f0729d4\n\t", "DUALANTENNAHEADINGA,USB3,0,51.0,FINESTEERING,2107,282205.000,02000000,d426,15824;INSUFFICIENT_OBS,NONE,0.000000000,0.000000000,0.000000000,0.0,0.000000000,0.000000000,\"\",0,0,0,0,00,00,00,00*a6944ad3\n\t", "INSPVAXA,USB3,0,53.0,FINESTEERING,2107,282205.550,02000000,471d,15824;INS_ALIGNMENT_COMPLETE,INS_RTKFIXED,37.37080836161,126.72396276793,9.6416,22.3000,-0.1860,0.2071,0.0131,-0.386237620,1.395044510,120.415786575,0.4755,0.3044,0.5933,0.1227,0.0990,0.0774,0.1450,0.1497,4.9912,0f000001,0*671127a5\n\t", "DUALANTENNAHEADINGA,USB3,0,53.0,FINESTEERING,2107,282206.000,02000000,d426,15824;INSUFFICIENT_OBS,NONE,0.000000000,0.000000000,0.000000000,0.0,0.000000000,0.000000000,\"\",0,0,0,0,00,00,00,00*e9703f6f\n\t", "INSPVAXA,USB3,0,52.0,FINESTEERING,2107,282207.050,02000000,471d,15824;INS_ALIGNMENT_COMPLETE,INS_RTKFIXED,37.37080624605,126.72396663060,9.6483,22.3000,-0.1799,0.2155,-0.0033,-0.382267918,1.666666307,118.913486054,0.4622,0.2990,0.5698,0.1222,0.0981,0.0770,0.1443,0.1494,4.9912,0f000001,0*412cbbed\n\t", "INSPVAXA,USB3,0,52.5,FINESTEERING,2107,282207.550,02000000,471d,15824;INS_ALIGNMENT_COMPLETE,INS_RTKFIXED,37.37080553452,126.72396795365,9.6521,22.3000,-0.1872,0.2206,-0.0051,-0.332963269,1.523153610,118.680008658,0.4622,0.2990,0.5698,0.1222,0.0981,0.0770,0.1443,0.1494,4.9912,0f000001,0*ceea6f3f\n\t", "DUALANTENNAHEADINGA,USB3,0,52.5,FINESTEERING,2107,282208.000,02000000,d426,15824;INSUFFICIENT_OBS,NONE,0.000000000,0.000000000,0.000000000,0.0,0.000000000,0.000000000,\"\",0,0,0,0,00,00,00,00*6ec42887\n\t", "DUALANTENNAHEADINGA,USB3,0,53.0,FINESTEERING,2107,282209.500,02000000,d426,15824;SOL_COMPUTED,L1_FLOAT,-1.000000000,126.771110535,-42.657562256,0.0,360.000000000,180.000000000,\"631T\",15,6,6,5,04,00,20,03*5e6f8f1e\n\t", "INSPVAXA,USB3,0,46.5,FINESTEERING,2107,282210.550,02000000,471d,15824;INS_ALIGNMENT_COMPLETE,INS_RTKFIXED,37.37080130132,126.72397594412,9.6761,22.3000,-0.1788,0.2268,0.0030,-0.286685420,1.503985922,118.659616564,0.4924,0.3183,0.5916,0.1238,0.0973,0.0785,0.1441,0.1495,4.9922,0f000001,0*a986a7a1\n\t", "INSPVAXA,USB3,0,46.5,FINESTEERING,2107,282211.050,02000000,471d,15824;INS_ALIGNMENT_COMPLETE,INS_RTKFIXED,37.37080065460,126.72397731700,9.6819,22.3000,-0.1828,0.2291,0.0069,-0.471563317,1.301185162,118.765096011,0.4785,0.3076,0.5799,0.1215,0.0954,0.0779,0.1439,0.1491,4.9928,0f000001,0*2dcee279\n\t", "INSPVAXA,USB3,0,49.5,FINESTEERING,2107,282211.550,02000000,471d,15824;INS_ALIGNMENT_COMPLETE,INS_RTKFIXED,37.37079998486,126.72397867623,9.6862,22.3000,-0.1762,0.2152,0.0021,-0.525326899,1.337901633,118.895801631,0.4785,0.3076,0.5799,0.1215,0.0954,0.0779,0.1439,0.1491,4.9928,0f000001,0*f623f6b1\n\t", "INSPVAXA,USB3,0,48.0,FINESTEERING,2107,282212.550,02000000,471d,15824;INS_ALIGNMENT_COMPLETE,INS_RTKFIXED,37.37079858565,126.72398137805,9.6949,22.3000,-0.1865,0.2376,0.0037,-0.452411122,1.244077399,119.281089900,0.4696,0.3015,0.5709,0.1202,0.0946,0.0776,0.1439,0.1489,4.9934,0f000001,0*f2809ec3\n\t", "INSPVAXA,USB3,0,48.0,FINESTEERING,2107,282213.050,02000000,471d,15824;INS_ALIGNMENT_COMPLETE,INS_RTKFIXED,37.37079782312,126.72398277607,9.6996,22.3000,-0.1874,0.2360,0.0136,-0.341636601,1.253165011,119.484687507,0.4696,0.3015,0.5709,0.1202,0.0946,0.0776,0.1439,0.1489,4.9934,0f000001,0*32ae8dd5\n\t", "INSPVAXA,USB3,0,52.0,FINESTEERING,2107,282213.550,02000000,471d,15824;INS_ALIGNMENT_COMPLETE,INS_RTKFIXED,37.37079696943,126.72398406821,9.7061,22.3000,-0.1973,0.2288,0.0187,-0.230921805,1.180153263,119.768927864,0.4696,0.3015,0.5709,0.1202,0.0946,0.0776,0.1439,0.1489,4.9934,0f000001,0*21be5dd7\n\t", "INSPVAXA,USB3,0,52.0,FINESTEERING,2107,282214.050,02000000,471d,15824;INS_ALIGNMENT_COMPLETE,INS_RTKFIXED,37.37079609402,126.72398538509,9.7128,22.3000,-0.1984,0.2265,0.0093,-0.318894921,1.159811562,120.132243890,0.4696,0.3015,0.5709,0.1202,0.0946,0.0776,0.1439,0.1489,4.9934,0f000001,0*fc389eb4\n\t", "INSPVAXA,USB3,0,52.0,FINESTEERING,2107,282215.050,02000000,471d,15824;INS_ALIGNMENT_COMPLETE,INS_RTKFIXED,37.37079433087,126.72398790668,9.7264,22.3000,-0.2059,0.2196,0.0017,-0.257763882,1.185688863,120.911498528,0.5642,0.3665,0.6560,0.1320,0.1043,0.0817,0.1458,0.1507,4.9969,0f000001,0*cb6b0c5a\n\t", "INSPVAXA,USB3,0,51.0,FINESTEERING,2107,282215.550,02000000,471d,15824;INS_ALIGNMENT_COMPLETE,INS_RTKFIXED,37.37079367366,126.72398934399,9.7308,22.3000,-0.1996,0.2242,0.0120,-0.145309566,1.145371194,121.351414848,0.5642,0.3665,0.6560,0.1320,0.1043,0.0817,0.1458,0.1507,4.9969,0f000001,0*eab453aa\n\t", "INSPVAXA,USB3,0,50.0,FINESTEERING,2107,282216.050,02008000,471d,15824;INS_ALIGNMENT_COMPLETE,INS_RTKFIXED,37.37079301498,126.72399074721,9.7351,22.3000,-0.2016,0.2239,0.0141,-0.200785279,1.162503620,121.722794866,0.5181,0.3306,0.6284,0.1253,0.0993,0.0793,0.1452,0.1498,4.9985,0f000001,0*bb6b6e1a\n\t", "INSPVAXA,USB3,0,50.0,FINESTEERING,2107,282216.550,02008000,471d,15824;INS_ALIGNMENT_COMPLETE,INS_RTKFIXED,37.37079227472,126.72399206413,9.7382,22.3000,-0.1946,0.2230,0.0198,-0.317684959,1.282586608,122.063744608,0.5181,0.3306,0.6284,0.1253,0.0993,0.0793,0.1452,0.1498,4.9985,0f000001,0*e6f737e3\n\t", "INSPVAXA,USB3,0,50.0,FINESTEERING,2107,282217.050,02008000,471d,15824;INS_ALIGNMENT_COMPLETE,INS_RTKFIXED,37.37079150006,126.72399338506,9.7418,22.3000,-0.1973,0.2143,0.0166,-0.258493900,1.347892765,122.299122592,0.4919,0.3126,0.6073,0.1228,0.0982,0.0779,0.1450,0.1495,4.9999,0f000001,0*de2ea87f\n\t", "INSPVAXA,USB3,0,51.5,FINESTEERING,2107,282218.550,02008000,471d,15824;INS_ALIGNMENT_COMPLETE,INS_RTKFIXED,37.37078915904,126.72399716309,9.7610,22.3000,-0.2130,0.2098,0.0170,-0.292581924,1.665037995,123.167578818,0.4769,0.3037,0.5912,0.1221,0.0981,0.0771,0.1448,0.1493,5.0010,0f000001,0*5a89842f\n\t", "INSPVAXA,USB3,0,51.5,FINESTEERING,2107,282219.050,02008000,471d,15824;INS_ALIGNMENT_COMPLETE,INS_RTKFIXED,37.37078832063,126.72399842807,9.7659,22.3000,-0.2077,0.2129,0.0166,-0.240249053,1.576876220,123.403306266,0.4687,0.2996,0.5787,0.1217,0.0981,0.0767,0.1445,0.1492,5.0017,0f000001,0*d445f717\n\t", "INSPVAXA,USB3,0,52.5,FINESTEERING,2107,282219.550,02008000,471d,15824;INS_ALIGNMENT_COMPLETE,INS_RTKFIXED,37.37078751914,126.72399965144,9.7712,22.3000,-0.2065,0.2085,0.0140,-0.281116396,1.447393421,123.657865027,0.4687,0.2996,0.5787,0.1217,0.0981,0.0767,0.1445,0.1492,5.0017,0f000001,0*13bb7dd6\n\t", "INSPVAXA,USB3,0,52.5,FINESTEERING,2107,282220.050,02008000,471d,15824;INS_ALIGNMENT_COMPLETE,INS_RTKFIXED,37.37078669426,126.72400086844,9.7773,22.3000,-0.1998,0.2016,0.0200,-0.389870934,1.544632790,123.892841428,0.4687,0.2996,0.5787,0.1217,0.0981,0.0767,0.1445,0.1492,5.0017,0f000001,0*0724934d\n\t", "INSPVAXA,USB3,0,45.0,FINESTEERING,2107,282220.550,02000000,471d,15824;INS_ALIGNMENT_COMPLETE,INS_RTKFIXED,37.37078572061,126.72400205426,9.7874,22.3000,-0.2160,0.2146,0.0148,-0.304638903,1.496803288,124.054451305,0.4687,0.2996,0.5787,0.1217,0.0981,0.0767,0.1445,0.1492,5.0017,0f000001,0*4ea05ecc\n\t", "INSPVAXA,USB3,0,45.0,FINESTEERING,2107,282221.050,02000000,471d,15824;INS_ALIGNMENT_COMPLETE,INS_RTKFIXED,37.37078472745,126.72400323556,9.7963,22.3000,-0.2252,0.2194,0.0154,-0.213568919,1.398343739,124.133980325,0.4687,0.2996,0.5787,0.1217,0.0981,0.0767,0.1445,0.1492,5.0017,0f000001,0*532042ec\n\t", "INSPVAXA,USB3,0,51.5,FINESTEERING,2107,282221.550,02000000,471d,15824;INS_ALIGNMENT_COMPLETE,INS_RTKFIXED,37.37078368778,126.72400445240,9.8057,22.3000,-0.2341,0.2209,0.0324,-0.018062526,1.300633595,124.151210863,0.4687,0.2996,0.5787,0.1217,0.0981,0.0767,0.1445,0.1492,5.0017,0f000001,0*d5cded7b\n\t", "INSPVAXA,USB3,0,51.5,FINESTEERING,2107,282222.050,02000000,471d,15824;INS_ALIGNMENT_COMPLETE,INS_RTKFIXED,37.37078266162,126.72400570863,9.8159,22.3000,-0.2293,0.2203,0.0286,-0.177364447,1.182183127,124.095380159,0.5655,0.3677,0.6592,0.1343,0.1069,0.0811,0.1457,0.1508,5.0028,0f000001,0*1d515c3b\n\t", "INSPVAXA,USB3,0,52.0,FINESTEERING,2107,282222.550,02000000,471d,15824;INS_ALIGNMENT_COMPLETE,INS_RTKFIXED,37.37078201526,126.72400713650,9.8181,22.3000,-0.2189,0.2044,0.0167,-0.239686925,1.045245044,123.863741135,0.5655,0.3677,0.6592,0.1343,0.1069,0.0811,0.1457,0.1508,5.0028,0f000001,0*9d8dd707\n\t", "INSPVAXA,USB3,0,52.0,FINESTEERING,2107,282223.050,02000000,471d,15824;INS_ALIGNMENT_COMPLETE,INS_RTKFIXED,37.37078138218,126.72400846731,9.8199,22.3000,-0.2177,0.1996,0.0188,-0.144202843,1.121525384,123.301599310,0.5655,0.3677,0.6592,0.1343,0.1069,0.0811,0.1457,0.1508,5.0028,0f000001,0*4658464e\n\t", "INSPVAXA,USB3,0,52.0,FINESTEERING,2107,282223.550,02000000,471d,15824;INS_ALIGNMENT_COMPLETE,INS_RTKFIXED,37.37078042542,126.72400959885,9.8298,22.3000,-0.1980,0.1883,0.0199,0.083241737,1.323181933,122.442356839,0.5655,0.3677,0.6592,0.1343,0.1069,0.0811,0.1457,0.1508,5.0028,0f000001,0*8c550850\n\t", "INSPVAXA,USB3,0,52.0,FINESTEERING,2107,282224.050,02000000,471d,15824;INS_ALIGNMENT_COMPLETE,INS_RTKFIXED,37.37077948836,126.72401076262,9.8410,22.3000,-0.2038,0.2000,0.0255,0.037457122,1.616174410,121.334966329,0.5655,0.3677,0.6592,0.1343,0.1069,0.0811,0.1457,0.1508,5.0028,0f000001,0*1dc4c535\n\t", "INSPVAXA,USB3,0,53.0,FINESTEERING,2107,282224.550,02000000,471d,15824;INS_ALIGNMENT_COMPLETE,INS_RTKFIXED,37.37077854921,126.72401195388,9.8525,22.3000,-0.2034,0.2018,0.0231,0.005685639,1.610626959,120.264541243,0.5655,0.3677,0.6592,0.1343,0.1069,0.0811,0.1457,0.1508,5.0028,0f000001,0*90090751\n\t", "INSPVAXA,USB3,0,53.0,FINESTEERING,2107,282225.050,02000000,471d,15824;INS_ALIGNMENT_COMPLETE,
